vi "Record Found.vi"(2 "Record":T1, 8 "error in (no error)":errorcluster, 11 "Car Wash Controller in":refnum<class "Car Wash Controller.lvclass">) -> (0 "error out":errorcluster, 3 "Car Wash Controller out":refnum<class "Car Wash Controller.lvclass">)   [LabVIEW 2012, in "Car Wash Controller.lvlib" / "Car Wash Controller.lvclass"]
uses:
  Car Wash Controller.lvclass
  Configuration Database API/Configuration Database API/Record.ctl
  Configuration Database API/Configuration Database API/Configuration Database API.lvclass
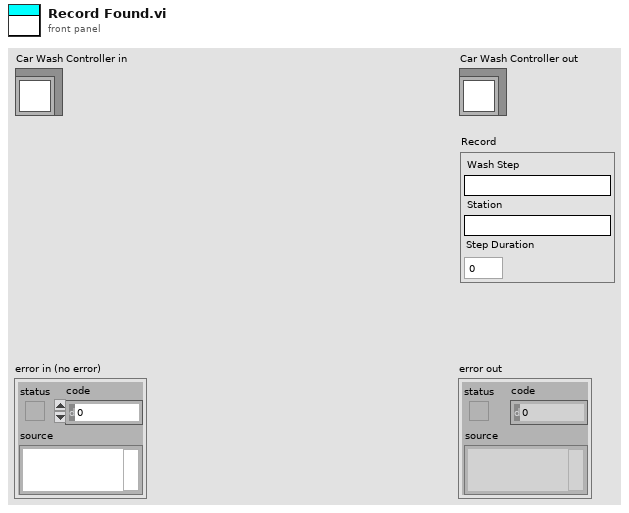
[diagram p1: front panel]
types:
  T1 = typedef "Configuration Database API.lvlib/Configuration Database API.lvclass/Record.ctl" = cluster{"Wash Step":string, "Station":string, "Step Duration":u8}
  T2 = typedef "Car Wash Controller.lvlib/Car Wash Controller.lvclass/Car Wash Controller State.ctl" = enum16{"Initial State", "Wait For Start State", "Start State", "Wait For Vehicle Position State", "Wash Step Execution State", "Wash Step / Cycle Completion State", "Wash Exit State", "Wash Abort / Terminate State"}
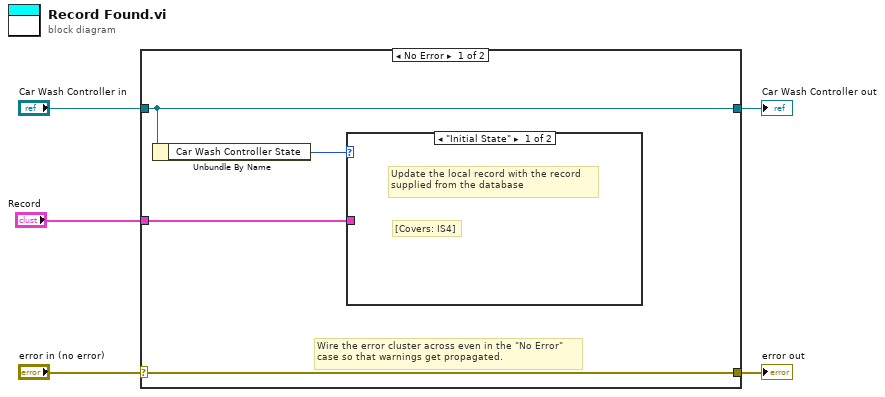
[diagram p0: block diagram]
diagram:
  n1 = case shown="No Error" "error in (no error)" {
    selector: "error in (no error)" -> [w9 w11]
    tunnel: [w9 w11] -> w4
    tunnel: [w8 w10] -> w2
    tunnel: "Car Wash Controller in" -> [w8 w10]
    tunnel: "Record" -> [w6 _]
    frame No Error {
      # "Wire the error cluster across even in the \"No Error\"\ncase so that warnings get propagated."
      n2 = Unbundle By Name(w8) -> ("Car Wash Controller State"=w7:T2)
      n3 = case shown="\"Initial State\"" w7 {
        tunnel: w6 -> [_ _]
        frame "Initial State" {
          # "[Covers: IS4]"
          # "Update the local record with the record\nsupplied from the database"
        }
        frame "Wait For Start State" {
        }
      }
    }
    frame Error {
    }
  }
  "error out" <- w4
  "Car Wash Controller out" <- w2
